vi "SM_Kolmogan.vi"() -> ()   [LabVIEW 2019, in "Kolmogan Library 1.lvlib"]
uses:
  Kolmogan Library 1.lvlib
panel:
  in  "等候秒數 4":i32=15
  out "End time 4":timestamp=timestamp(3742957067.58093 s since 1904-01-01)
  out "current time 4":timestamp=timestamp(3742957049.546739 s since 1904-01-01)
  out "current time 3":timestamp=timestamp(3742956976.4306865 s since 1904-01-01)
  out "current time 2":timestamp=timestamp(3742956973.4187617 s since 1904-01-01)
  in  "等候秒數 2":i32=10
  in  "等候秒數 3":i32=10
  out "剩餘秒數 4":i32=5
  out "等候逾時 4":bool
  out "Error status 4":bool
  out "移動完成 4":bool=TRUE
  out "剩餘秒數 2":i32=5
  out "等候逾時 2":bool
  out "Error status 2":bool
  out "等待觸發":bool=TRUE
  out "找到原點":bool=TRUE
  out "State machine":i32=4
  out "螺絲檢測結果":string="檢測完成"
  in  "Trigger":u16(ring) items=["等待觸發", "觸發拍攝"]
  out "剩餘秒數 3":i32=9
  out "等候逾時 3":bool
  out "Error status 3":bool
  out "移動完成 3":bool=TRUE
  out "Motion State":bool[](array[boolean])=[FALSE, TRUE, TRUE, FALSE, FALSE, FALSE, FALSE, FALSE, FALSE, FALSE, FALSE, TRUE, FALSE, FALSE, FALSE, TRUE, FALSE, FALSE, FALSE, FALSE, FALSE, FALSE, FALSE, FALSE, FALSE, FALSE, FALSE, FALSE, FALSE, FALSE, FALSE, FALSE]
  in  "IP:Port":string="192.168.1.11:502"
  # "State machine (等待觸發燈號)\n1. 建立連線\n2. 復歸 [ SW(F), Camera(F) ]\n3. 找原點 (Home position found)\n4. 初始位置 (15)\n5. 等待觸發 (確認有在原點)\n>>相機\n>>掃描 (15)\n>>復歸 [ SW(F), Camera(F) ]\n6. 取值\n7. Error 重新建立連線"
  # "#588 959/1174 這邊要問Andy"
  # "#268 600/1174 State"
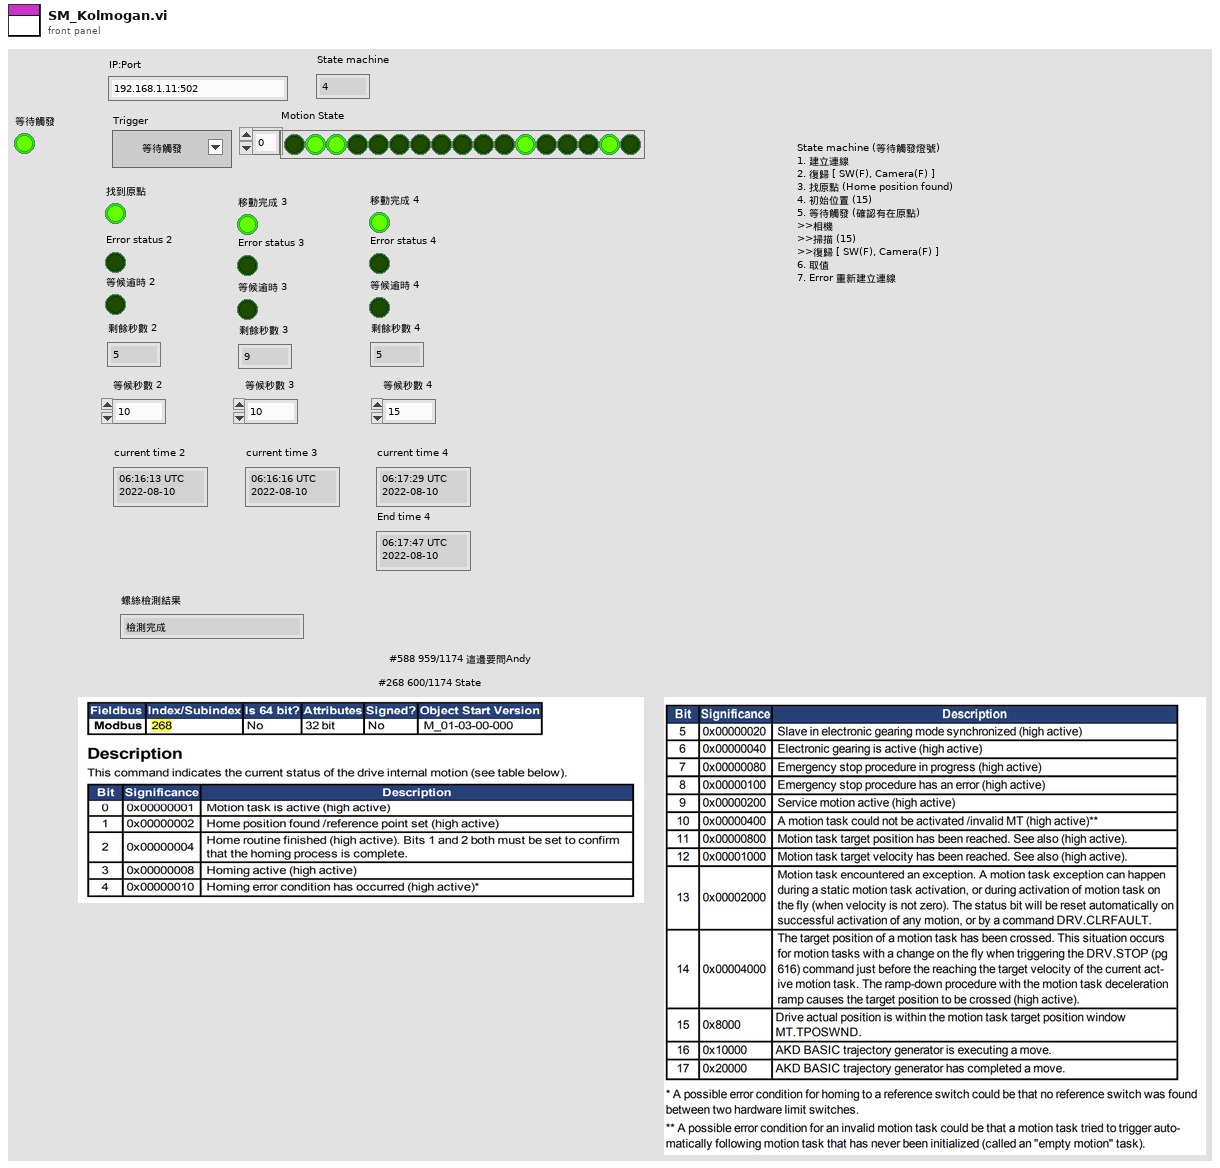
[diagram p1: front panel]
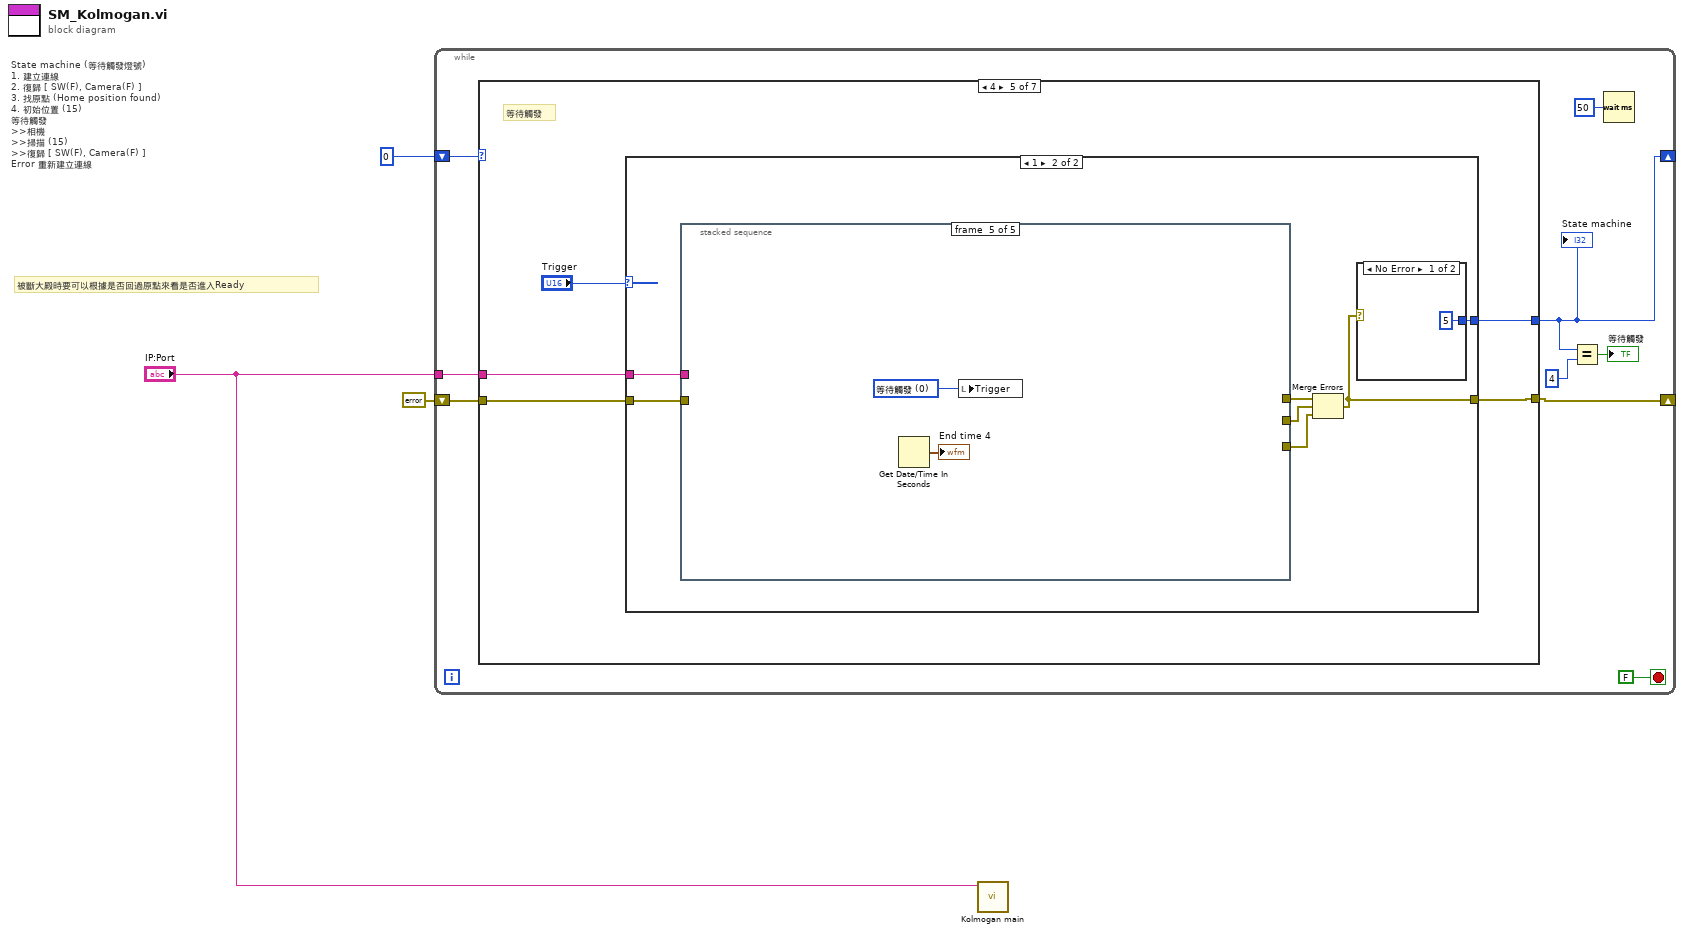
[diagram p0: block diagram]
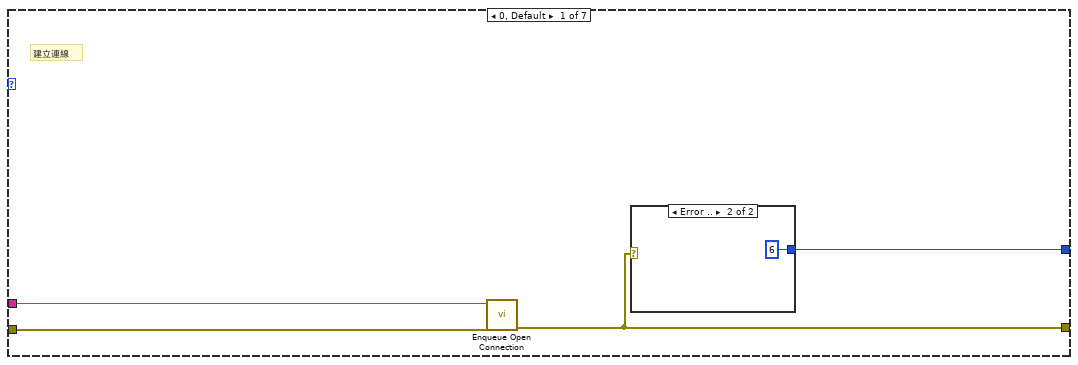
[diagram p2: hidden frame]
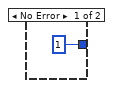
[diagram p3: hidden frame]
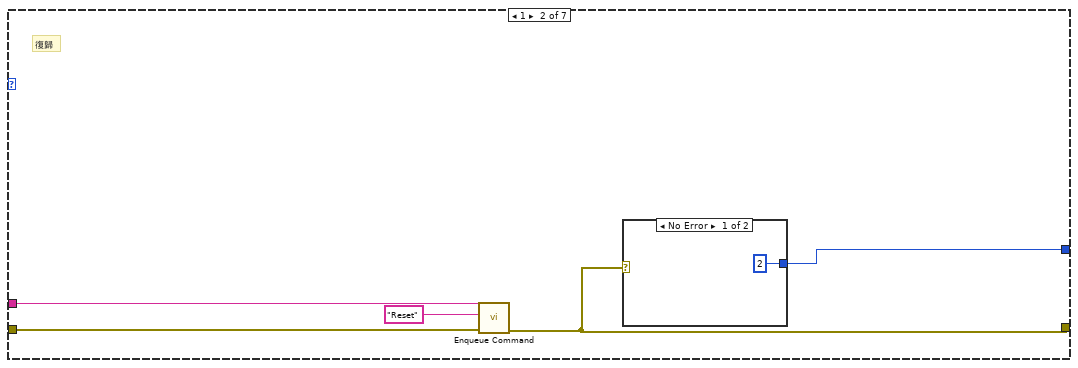
[diagram p4: hidden frame]
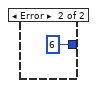
[diagram p5: hidden frame]
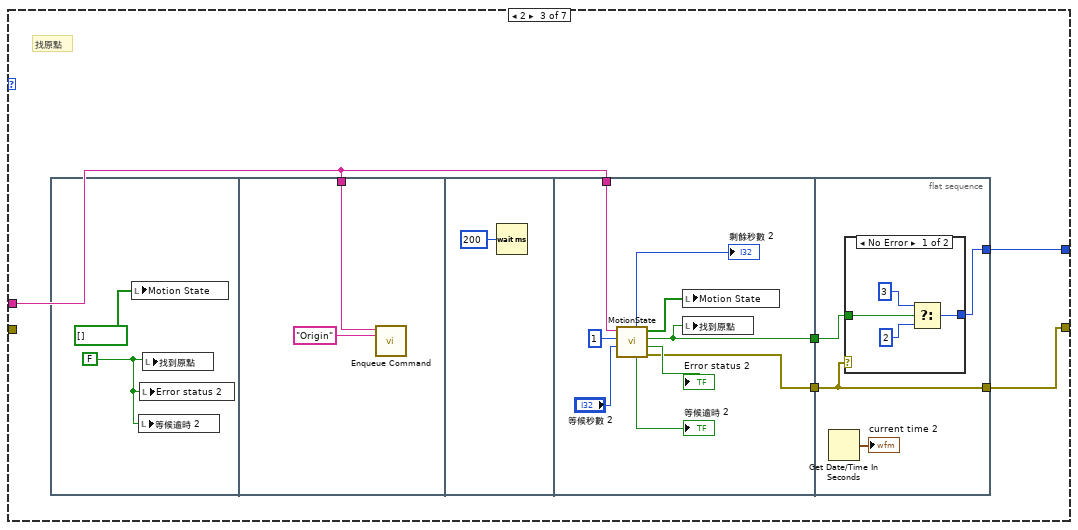
[diagram p6: hidden frame]
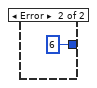
[diagram p7: hidden frame]
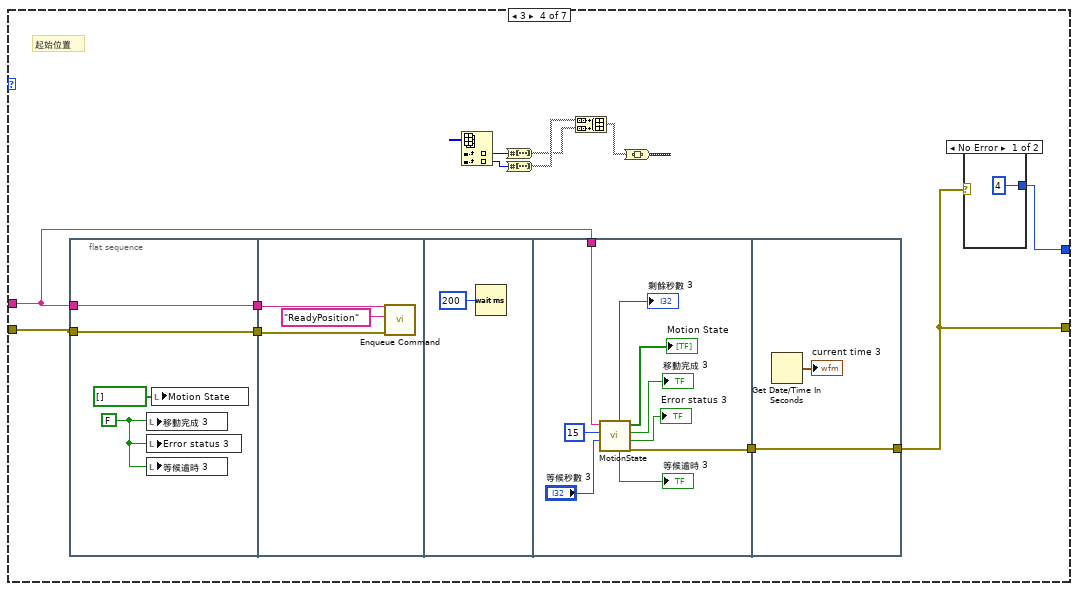
[diagram p8: hidden frame]
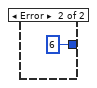
[diagram p9: hidden frame]
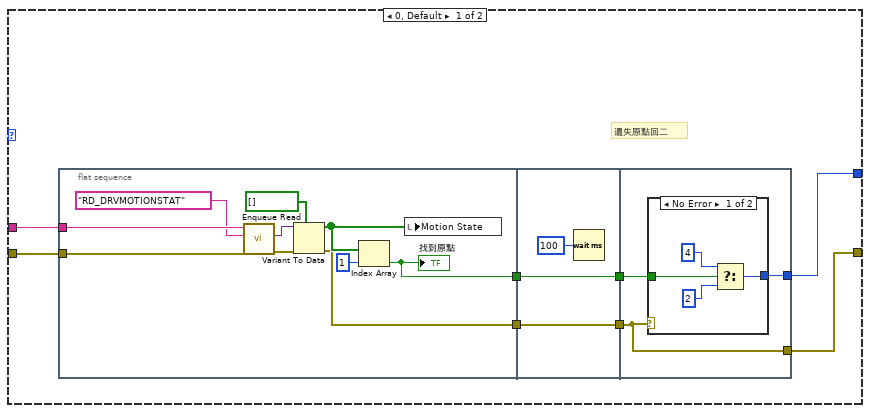
[diagram p10: hidden frame]
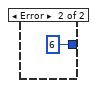
[diagram p11: hidden frame]
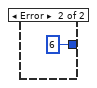
[diagram p12: hidden frame]
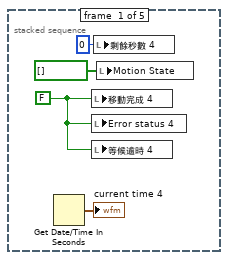
[diagram p13: hidden frame]
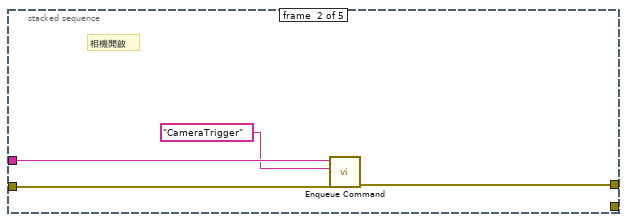
[diagram p14: hidden frame]
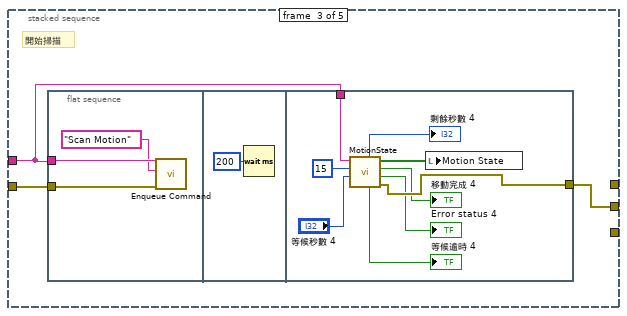
[diagram p15: hidden frame]
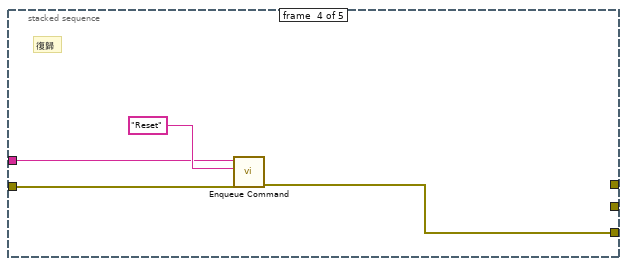
[diagram p16: hidden frame]
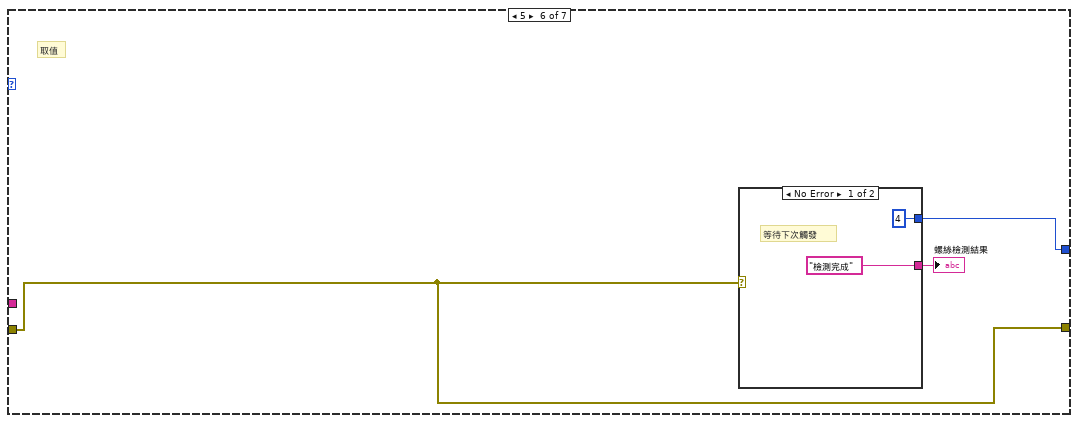
[diagram p17: hidden frame]
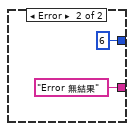
[diagram p18: hidden frame]
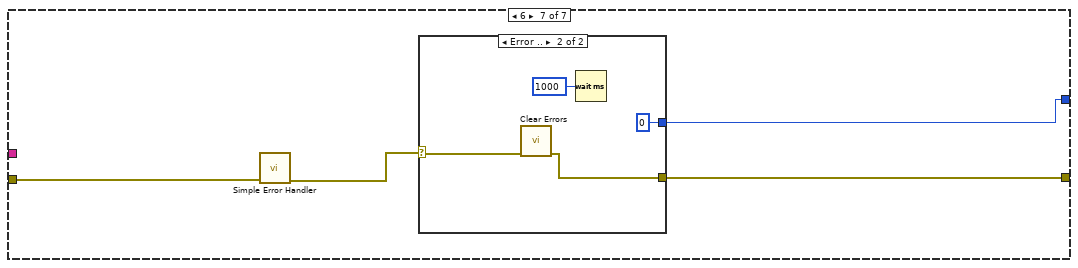
[diagram p19: hidden frame]
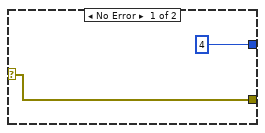
[diagram p20: hidden frame]
diagram:
  # "被斷大殿時要可以根據是否回過原點來看是否進入Ready"
  # "State machine (等待觸發燈號)\n1. 建立連線\n2. 復歸 [ SW(F), Camera(F) ]\n3. 找原點 (Home position found)\n4. 初始位置 (15)\n等待觸發\n>>相機\n>>掃描 (15)\n>>復歸 [ SW(F), Camera(F) ]\nError 重新建立連線"
  n1 = while {
    tunnel: "IP:Port" -> [w11]
    shift-right: [w10] -> _
    shift-left: errorcluster {"status"=FALSE, "code"=0, "source"=""} ("Error Out") -> [w9]
    shift-right: [w7] -> _
    shift-left: 0 -> [w12]
    stop <- FALSE stop-if-true
    n2 = case shown="4" w12 {
      tunnel: w11 -> [w16 w21 w30 w58 w84 _ _]
      tunnel: [w14 w20 w29 w57 w82 w156 w163] -> w10
      tunnel: w9 -> [w15 w22 _ w60 w83 w156 w165]
      tunnel: [w13 w19 w26 w59 w85 w155 w162] -> w7
      frame 0, Default {
        # "建立連線"
        n3 = call "Enqueue Open Connection.vi"("Error In"=w15, "Name"=w16) -> ("Error Out"=w14:errorcluster)  [unwired: 9 in]
        n4 = case shown="Error .." w14 {
          tunnel: [1 6] -> w13
          frame No Error {
          }
          frame Error {
          }
        }
      }
      frame 1 {
        # "復歸"
        n5 = call "Enqueue Command.vi"("Error In"=w22, "Message"="Reset", "Name"=w21) -> ("Error Out"=w20:errorcluster)  [unwired: 8 in]
        n6 = case shown="No Error" w20 {
          tunnel: [2 6] -> w19
          frame No Error {
          }
          frame Error {
          }
        }
      }
      frame 2 {
        # "找原點"
        n7 = flat-sequence {
          tunnel: w30 -> [w34]
          tunnel: w30 -> [w42]
          tunnel: [w37] -> w28
          tunnel: [w36] -> w27
          tunnel: [w45] -> w29
          tunnel: w28 -> [w45]
          tunnel: w27 -> [w47]
          tunnel: [w46] -> w26
          frame #0 {
            w32 = FALSE ("移動完成")
            n8 = local write "Motion State"(bool[] [] ("Motion State")) -> ()
            n9 = local write "等候逾時 2"(w32) -> ()
            n10 = local write "Error status 2"(w32) -> ()
            n11 = local write "找到原點"(w32) -> ()
          }
          frame #1 {
            n12 = call "Enqueue Command.vi"("Message"="Origin", "Name"=w34) -> ()  [unwired: 9 in, 1 out]
          }
          frame #2 {
            n13 = Wait (ms)(milliseconds to wait=u32 200) -> ()  [unwired: 1 out]
          }
          frame #3 {
            n14 = call "MotionState.vi"("等候秒數"="等候秒數 2", "index"=1, "IP:Port"=w42) -> ("error out"=w37:errorcluster, "Error status"=→"Error status 2":bool, "移動完成"=w36:bool, "Motion State"=w41:bool[], "等候逾時"=→"等候逾時 2":bool, "剩餘秒數"=→"剩餘秒數 2":i32)  [unwired: 3 in]
            n15 = local write "Motion State"(w41) -> ()
            n16 = local write "找到原點"(w36) -> ()
          }
          frame #4 {
            n17 = Get Date/Time In Seconds() -> (seconds since 1Jan1904=→"current time 2":timestamp)
            n18 = case shown="No Error" w45 {
              tunnel: w47 -> [w52 _]
              tunnel: [w49 6 ("f")] -> w46
              frame No Error {
                n19 = Select(t=3, s=w52, f=2) -> (s? t:f=w49:i32)
              }
              frame Error {
              }
            }
          }
        }
      }
      frame 3 {
        # "起始位置"
        n20 = flat-sequence {
          tunnel: w58 -> [w63]
          tunnel: w60 -> [w64]
          tunnel: [w64] -> w56
          tunnel: [w63] -> w55
          tunnel: w56 -> [w66]
          tunnel: w55 -> [w65]
          tunnel: w58 -> [w77]
          tunnel: [w76] -> w54
          tunnel: [w79] -> w57
          tunnel: w54 -> [w79]
          frame #0 {
            w61 = FALSE ("移動完成")
            n21 = local write "移動完成 3"(w61) -> ()
            n22 = local write "Error status 3"(w61) -> ()
            n23 = local write "等候逾時 3"(w61) -> ()
            n24 = local write "Motion State"(bool[] [] ("Motion State")) -> ()
          }
          frame #1 {
            n25 = call "Enqueue Command.vi"("Error In"=w66, "Message"="ReadyPosition", "Name"=w65) -> ()  [unwired: 8 in, 1 out]
          }
          frame #2 {
            n26 = Wait (ms)(milliseconds to wait=u32 200) -> ()  [unwired: 1 out]
          }
          frame #3 {
            n27 = call "MotionState.vi"("等候秒數"="等候秒數 3", "index"=15, "IP:Port"=w77) -> ("error out"=w76:errorcluster, "Error status"=→"Error status 3":bool, "移動完成"=→"移動完成 3":bool, "Motion State"=→"Motion State":bool[], "等候逾時"=→"等候逾時 3":bool, "剩餘秒數"=→"剩餘秒數 3":i32)  [unwired: 3 in]
          }
          frame #4 {
            n28 = Get Date/Time In Seconds() -> (seconds since 1Jan1904=→"current time 3":timestamp)
          }
        }
        n29 = case shown="No Error" w57 {
          tunnel: [4 6] -> w59
          frame No Error {
          }
          frame Error {
          }
        }
      }
      frame 4 {
        # "等待觸發"
        n30 = case shown="1" "Trigger" {
          tunnel: [w91 w117] -> w85
          tunnel: w84 -> [w94 w122]
          tunnel: w83 -> [w87 w121]
          tunnel: [w88 w116] -> w82
          frame 0, Default {
            # "遺失原點回二"
            n31 = flat-sequence {
              tunnel: w94 -> [w104]
              tunnel: [w97] -> w92
              tunnel: [w96] -> w89
              tunnel: w87 -> [w95]
              tunnel: [w106] -> w93
              tunnel: w92 -> [w106]
              tunnel: [w105] -> w90
              tunnel: w89 -> [w105]
              tunnel: w93 -> [w110]
              tunnel: [w109] -> w91
              tunnel: w90 -> [w108]
              tunnel: [w108] -> w88
              frame #0 {
                n32 = call "Enqueue Read.vi"("Error In"=w95, "Message"="RD_DRVMOTIONSTAT", "Name"=w104) -> ("Error Out"=w102:errorcluster, "Data"=w101:variant)  [unwired: 7 in]
                n33 = Variant To Data(error in=w102, type=bool[] [] ("appended array"), Variant=w101) -> (data=w98:bool[], error out=w96:errorcluster)
                n34 = Index Array(array=w98, index=1) -> (element=w97:bool)
                "找到原點" <- w97
                n35 = local write "Motion State"(w98) -> ()
              }
              frame #1 {
                n36 = Wait (ms)(milliseconds to wait=u32 100) -> ()  [unwired: 1 out]
              }
              frame #2 {
                n37 = case shown="No Error" w108 {
                  tunnel: w110 -> [w114 _]
                  tunnel: [w111 6 ("f")] -> w109
                  frame No Error {
                    n38 = Select(t=4, s=w114, f=2) -> (s? t:f=w111:i32)
                  }
                  frame Error {
                  }
                }
              }
            }
          }
          frame 1 {
            n39 = stacked-sequence {
              tunnel: w122 -> [_ w132 w134 w151 _]
              tunnel: w121 -> [_ w130 w135 w150 _]
              tunnel: [_ w129 _ _ _] -> w120
              tunnel: [_ _ w133 _ _] -> w119
              tunnel: [_ _ _ w149 _] -> w118
              frame #0 {
                w126 = FALSE ("移動完成")
                n40 = Get Date/Time In Seconds() -> (seconds since 1Jan1904=→"current time 4":timestamp)
                n41 = local write "移動完成 4"(w126) -> ()
                n42 = local write "Error status 4"(w126) -> ()
                n43 = local write "等候逾時 4"(w126) -> ()
                n44 = local write "剩餘秒數 4"(0 ("剩餘秒數")) -> ()
                n45 = local write "Motion State"(bool[] [] ("Motion State")) -> ()
              }
              frame #1 {
                # "相機開啟"
                n46 = call "Enqueue Command.vi"("Error In"=w130, "Message"="CameraTrigger", "Name"=w132) -> ("Error Out"=w129:errorcluster)  [unwired: 8 in]
              }
              frame #2 {
                # "開始掃描"
                n47 = flat-sequence {
                  tunnel: w135 -> [w138]
                  tunnel: w134 -> [w137]
                  tunnel: w134 -> [w148]
                  tunnel: [w146] -> w133
                  frame #0 {
                    n48 = call "Enqueue Command.vi"("Error In"=w138, "Message"="Scan Motion", "Name"=w137) -> ()  [unwired: 8 in, 1 out]
                  }
                  frame #1 {
                    n49 = Wait (ms)(milliseconds to wait=u32 200) -> ()  [unwired: 1 out]
                  }
                  frame #2 {
                    n50 = call "MotionState.vi"("等候秒數"="等候秒數 4", "index"=15, "IP:Port"=w148) -> ("error out"=w146:errorcluster, "Error status"=→"Error status 4":bool, "移動完成"=→"移動完成 4":bool, "Motion State"=w147:bool[], "等候逾時"=→"等候逾時 4":bool, "剩餘秒數"=→"剩餘秒數 4":i32)  [unwired: 3 in]
                    n51 = local write "Motion State"(w147) -> ()
                  }
                }
              }
              frame #3 {
                # "復歸"
                n52 = call "Enqueue Command.vi"("Error In"=w150, "Message"="Reset", "Name"=w151) -> ("Error Out"=w149:errorcluster)  [unwired: 8 in]
              }
              frame #4 {
                w154 = u16 0 items=["等待觸發", "觸發拍攝"] ("Menu Ring")
                n53 = Get Date/Time In Seconds() -> (seconds since 1Jan1904=→"End time 4":timestamp)
                n54 = local write "Trigger"(w154) -> ()
              }
            }
            n55 = Merge Errors(w120, w119, w118) -> (w116:errorcluster)
            n56 = case shown="No Error" w116 {
              tunnel: [5 6] -> w117
              frame No Error {
              }
              frame Error {
              }
            }
          }
        }
      }
      frame 5 {
        # "取值"
        n57 = case shown="No Error" w156 {
          tunnel: ["檢測完成" "Error 無結果"] -> w157
          tunnel: [4 6] -> w155
          frame No Error {
            # "等待下次觸發"
          }
          frame Error {
          }
        }
        "螺絲檢測結果" <- w157
      }
      frame 6 {
        n58 = call <vilib>:"Simple Error Handler.vi"("error in (no error)"=w165) -> ("error out"=w164:errorcluster)  [unwired: 4 in, 4 out]
        n59 = case shown="Error .." w164 {
          selector: w164 -> [w167 w171]
          tunnel: [w167 w169] -> w163
          tunnel: [4 0] -> w162
          frame No Error {
          }
          frame Error {
            n60 = call <vilib>:"Clear Errors.vi"("error in (no error)"=w171) -> ("error out"=w169:errorcluster)  [unwired: 5 in, 1 out]
            n61 = Wait (ms)(milliseconds to wait=u32 1000) -> ()  [unwired: 1 out]
          }
        }
      }
    }
    "State machine" <- w7
    n62 = Equal?(x=w7, y=4) -> (x = y?=→"等待觸發":bool)
    n63 = Wait (ms)(milliseconds to wait=u32 50) -> ()  [unwired: 1 out]
  }
  n64 = call "Kolmogan main.vi"("Name"="IP:Port") -> ()  [unwired: 10 in, 1 out]
